vi "Open.vi"(8 "error in (no error)":errorcluster, 11 "MyTestSuite in":refnum<class "MyTestSuite.lvclass">) -> (0 "error out":errorcluster, 3 "MyTestSuite out":refnum<class "MyTestSuite.lvclass">)   [LabVIEW 2020, in "MyTestSuite.lvclass"]
uses:
  MyTestSuite.lvclass
  MyTestSuite.lvclass/MyTestSuite.ctl
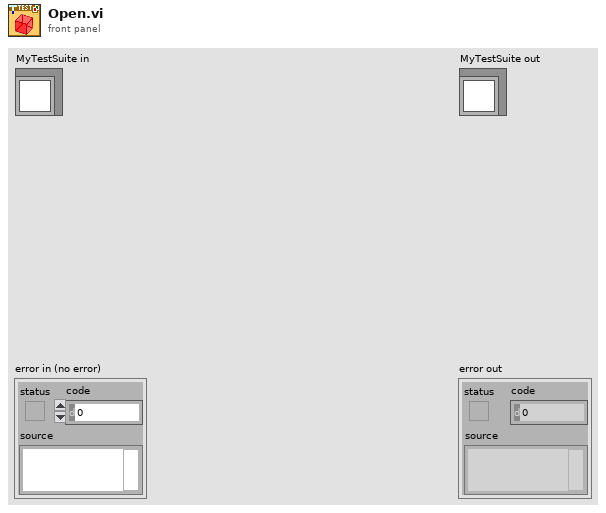
[diagram p1: front panel]
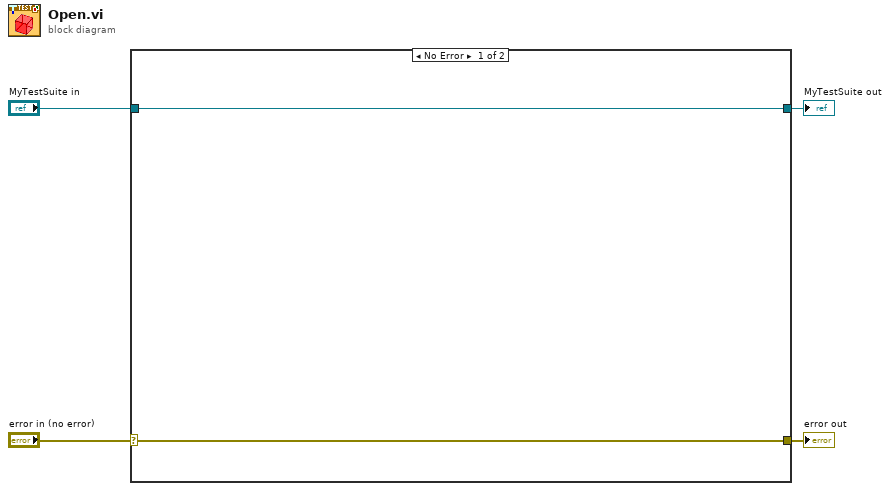
[diagram p0: block diagram]
diagram:
  n1 = case shown="No Error" "error in (no error)" {
    selector: "error in (no error)" -> [w5 w8]
    tunnel: [w5 w8] -> w3
    tunnel: [w6 w7] -> w1
    tunnel: "MyTestSuite in" -> [w6 w7]
    frame No Error {
    }
    frame Error {
    }
  }
  "error out" <- w3
  "MyTestSuite out" <- w1
